vi "Pre Launch Init.vi"(11 "Actor_log in":refnum<class "Actor_log.lvclass">) -> (0 "error out":errorcluster, 3 "Actor_log out":refnum<class "Actor_log.lvclass">)   [LabVIEW 2020, in "Actor_log.lvlib" / "Actor_log.lvclass"]
doc: "(<B>Filename</B>: Actor Framework.lvlib:Actor.lvclass:Pre Launch Init.vi)\n\nDefines behavior that occurs after the Launch Nested Actor method is invoked but before the actor's Actor Core method begins running.\n\nBy default, this method does nothing. A descendant class may override it to define behavior."
uses:
  Actor_log.lvclass
  Actor_log.lvclass/Actor_log.ctl
  <vilib>/ActorFramework/Actor/Actor.lvclass
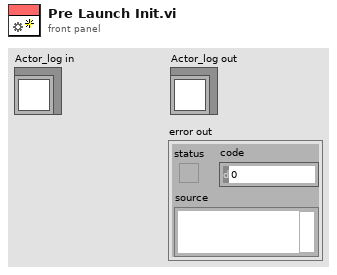
[diagram p1: front panel]
types:
  T1 = enum16{"open", "replace", "create", "open or create", "replace or create", "replace or create with confirmation"}
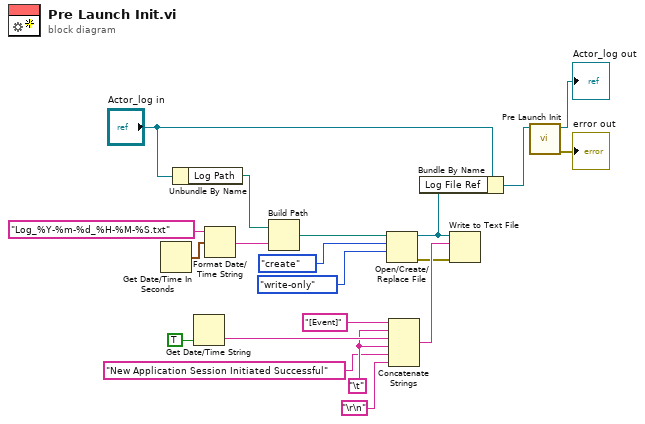
[diagram p0: block diagram]
diagram:
  w11 = "\t"
  n1 = Get Date/Time In Seconds() -> (seconds since 1Jan1904=w5:timestamp)
  n2 = Unbundle By Name("Actor_log in") -> ("Log Path"=w7:path)
  n3 = Get Date/Time String(want seconds? (F)=TRUE) -> (time string=w12:string)  [unwired: 2 in, 1 out]
  n4 = Format Date/Time String(time format string (%c)="Log_%Y-%m-%d_%H-%M-%S.txt", seconds (now)=w5) -> (date/time string=w3:string)  [unwired: 1 in]
  n5 = Build Path(base path=w7, name or relative path=w3) -> (appended path=w6:path)
  n6 = Open/Create/Replace File(file path (use dialog)=w6, operation (0:open)=T1."create", access (0:read/write)=enum16{"read/write", "read-only", "write-only"}."write-only") -> (refnum out=w1:refnum<file>, error out=w8:errorcluster)  [unwired: 3 in, 1 out]
  n7 = Concatenate Strings("[Event]" ("string"), w11, w12, w11, "New Application Session Initiated Successful" ("string"), "\r\n") -> (w9:string)
  n8 = Bundle By Name(cluster="Actor_log in", "Log File Ref"=w1) -> (w16:refnum<class "Actor_log.lvclass">)
  n9 = Write to Text File(file (use dialog)=w1, text=w9, error in=w8) -> ()  [unwired: 1 in, 3 out]
  n10 = call-parent "Pre Launch Init.vi"("Actor in"=w16) -> ("error out"=→"error out":errorcluster, "Actor out"=→"Actor_log out":refnum<class "Actor_log.lvclass">)  [unwired: 9 in]
